vi "Set Data Logging Rate (Target Rate).vi"(8 "error in (no error)":errorcluster, 11 "Data Logging Specification Ref in":T1) -> (0 "error out":errorcluster, 3 "Data Logging Specification Ref out":T1)   [LabVIEW 2020, in "NI_VS Data Logging API.lvlib"]
doc: "Specifies the rate at which to log data, in hertz. You can log at the rate at which the target produces data, or a custom rate. You must manually select the polymorphic instance to use."
uses:
  <vilib>/NI VeriStand/Execution/DataLogging/NI_VS Data Logging API.lvlib
  <vilib>/NI VeriStand/Execution/DataLogging/DataLoggingSpecification Ref.ctl
  NationalInstruments.VeriStand.ClientAPI
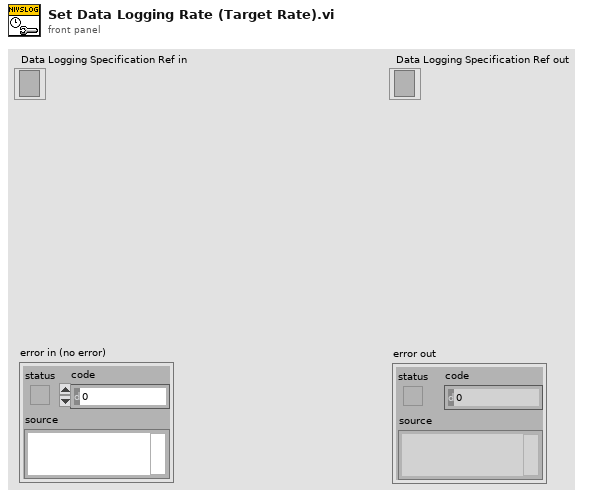
[diagram p1: front panel]
types:
  T1 = typedef "NI_VS Data Logging API.lvlib/DataLoggingSpecification Ref.ctl" = refnum<k24>
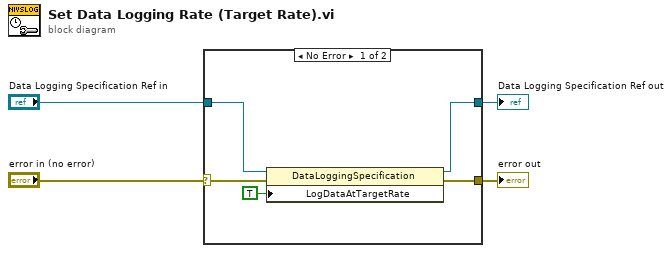
[diagram p0: block diagram]
diagram:
  n1 = case shown="No Error" "error in (no error)" {
    selector: "error in (no error)" -> [w9 w10]
    tunnel: "Data Logging Specification Ref in" -> [w8 w11]
    tunnel: [w7 w11] -> w2
    tunnel: [w6 w10] -> w1
    frame No Error {
      n2 = property class="DataLoggingSpecification"(reference=w8, error in=w9, "LogDataAtTargetRate"=TRUE) -> (reference out=w7:T1, error out=w6:errorcluster)
    }
    frame Error {
    }
  }
  "error out" <- w1
  "Data Logging Specification Ref out" <- w2
